vi "JSON text to Variant (path).vi"(7 "Item Path":string, 8 "error in (no error)":errorcluster, 9 "Variant (Data Type)":variant, 10 "Starting Offset":i32, 11 "JSON":string) -> (0 "error out":errorcluster, 1 "Variant out":variant, 3 "Found":bool)   [LabVIEW 2021, in "json.facade.lvlib"]
uses:
  json.facade.lvlib
  jsontext/JSONtext.lvlib
  jsontext/LVClass Serializer/JSONtext LVClass Serializer.lvclass
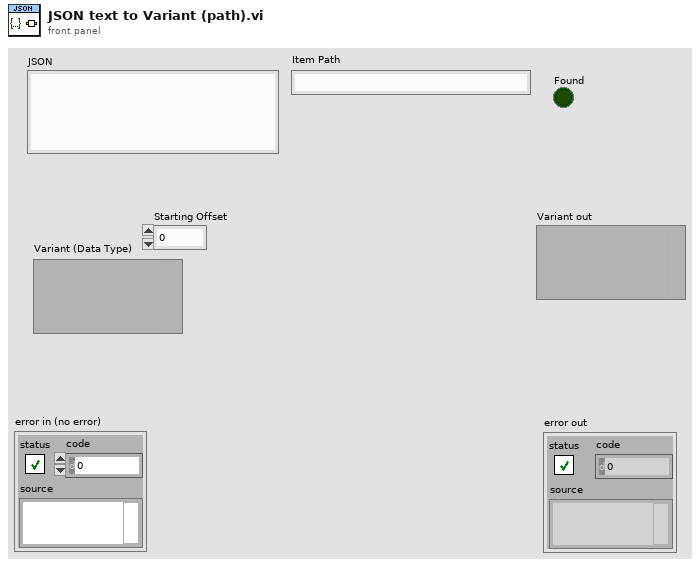
[diagram p1: front panel]
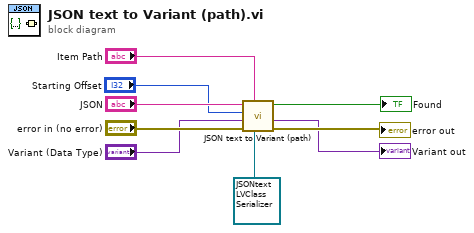
[diagram p0: block diagram]
diagram:
  n1 = call "JSON text to Variant (path).vi"("LVClass Serializer"=refnum<class "JSONtext LVClass Serializer.lvclass"> refnum, "Item $Path"="Item Path", "error in (no error)"="error in (no error)", "Variant (Data Type)"="Variant (Data Type)", "Starting Offset"="Starting Offset", "JSON"="JSON") -> ("error out"=→"error out":errorcluster, "Variant out"=→"Variant out":variant, "Found"=→"Found":bool)  [unwired: 3 in]
